vi "Get Package Info.vi"(11 "Selected Version":string) -> (0 "error out":errorcluster, 2 "URL":string, 3 "Build Date":timestamp format="%<%x %.3X>T")   [LabVIEW 2020, in "WebView2 Updater.lvclass"]
uses:
  WebView2 Updater.lvclass
  <vilib>/httpClient/LabVIEWHTTPClient.lvlib
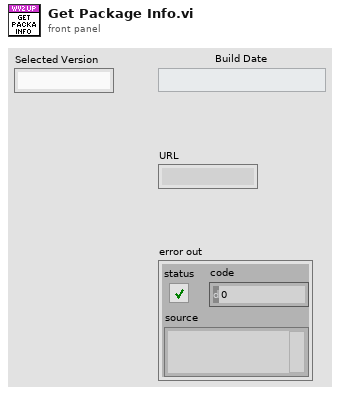
[diagram p1: front panel]
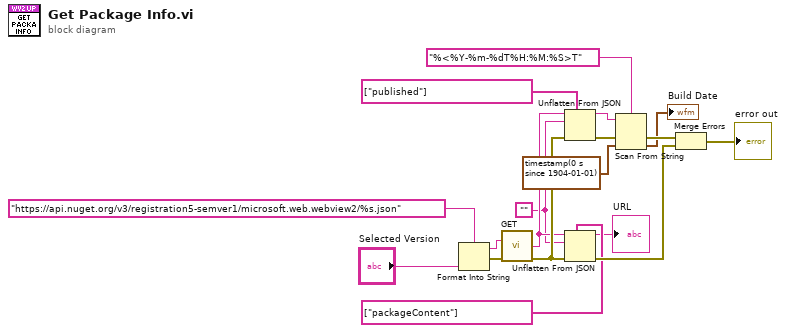
[diagram p0: block diagram]
diagram:
  w10 = ""
  n1 = Format Into String(format string="https://api.nuget.org/v3/registration5-semver1/microsoft.web.webview2/%s.json", "Selected Version") -> (resulting string=w11:string, error out=w12:errorcluster)  [unwired: 2 in]
  n2 = call <vilib>:"GET.vi"("url"=w11, "error in (no error)"=w12) -> ("body"=w15:string, "error out"=w16:errorcluster)  [unwired: 10 in, 2 out]
  n3 = Unflatten From JSON(path=string[] ["published"], JSON string=w15, type and defaults=w10, error in (no error)=w16) -> (value=w13:string, error out=w14:errorcluster)  [unwired: 3 in]
  n4 = Unflatten From JSON(path=string[] ["packageContent"], JSON string=w15, type and defaults=w10, error in (no error)=w16) -> (value=→"URL":string, error out=w18:errorcluster)  [unwired: 3 in]
  n5 = Scan From String(format string="%<%Y-%m-%dT%H:%M:%S>T", input string=w13, error in=w14, default 1=timestamp(0 s since 1904-01-01)) -> (error out=w17:errorcluster, output 1=→"Build Date":timestamp)  [unwired: 1 in, 2 out]
  n6 = Merge Errors(w17, w18) -> (→"error out":errorcluster)
